vi "PlumeCenterDetermination.vi"(7 "nPointsSampled":i32, 10 "SD Estimate":dbl, 11 "nPointsInRake":i32) -> (2 "CommandString":string, 3 "Measurement Center":dbl)   [LabVIEW 2011]
uses:
  GaussianGlobal.vi
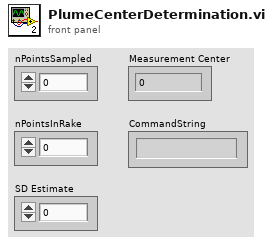
[diagram p1: front panel]
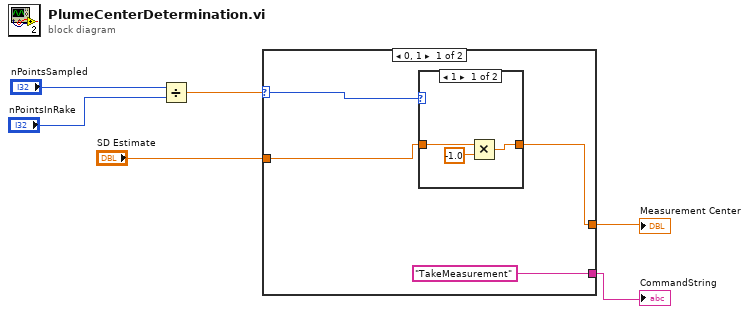
[diagram p0: block diagram]
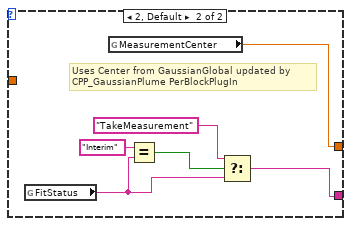
[diagram p3: hidden frame]
diagram:
  n1 = Divide(x="nPointsSampled", y="nPointsInRake") -> (x/y=w4:dbl)
  n2 = case shown="0, 1" w4 {
    selector: w4 -> [w10 _]
    tunnel: [w9 w20] -> w1
    tunnel: "SD Estimate" -> [w8 _]
    tunnel: ["TakeMeasurement" w15] -> w6
    frame 0, 1 {
      n3 = case shown="1" w10 {
        tunnel: w8 -> [w13 w14]
        tunnel: [w11 w14] -> w9
        frame 1 {
          n4 = Multiply(x=w13, y=-1.0) -> (x*y=w11:dbl)
        }
        frame 0, Default {
        }
      }
    }
    frame 2, Default {
      # "Uses Center from GaussianGlobal updated by\nCPP_GaussianPlume PerBlockPlugIn"
      n5 = global read "GaussianGlobal.vi" "FitStatus"() -> (w17:string)
      n6 = global read "GaussianGlobal.vi" "MeasurementCenter"() -> (w20:dbl)
      n7 = Equal?(x="Interim", y=w17) -> (x = y?=w18:bool)
      n8 = Select(t="TakeMeasurement", s=w18, f=w17) -> (s? t:f=w15:string)
    }
  }
  "CommandString" <- w6
  "Measurement Center" <- w1
